vi "TraverseDoAllChannels.vi"(0 "Current Pulses positions for all channels":sgl[](array[numeric]), 1 "Current Pos In Eng units of all channels":sgl[](array[numeric]) format="%.2f", 2 "Counters Reset?":bool, 5 "Backlash Compensation?":bool, 7 "Home":T1, 9 "Mode":T5, 11 "Position Steps":sgl[][](array[numeric]) format="%.2f", 12 "Matched Configurations all Channels In":T2[](array[typedef]) {"Static Drive Configuration"."Indexer Mode  (FSA)" items=["Incremental", "Absolute"]; "Static Drive Configuration"."Buffer at Stop (SSH)" items=["Clear buffer", "Save and Continue"]; "Static Drive Configuration"."Buffer at Limit (SSG)" items=["Clear buffer", "Save and Continue"]; "Static Drive Configuration"."RS232 Echo Control (SSA)" items=["Echo ON", "Echo OFF"]; "Static Drive Configuration"."Reference edge of Home (OSH)" items=["CW", "CCW"]; "Static Drive Configuration"."Encoder Z for Home (OSD)" items=["Don't use", "Enable"]; "Static Drive Configuration"."Home Switch Sense (OSC)" items=["Normally Open", "Normally Closed"]; "Static Drive Configuration"."Home Position (OSB)" items=["Anywhere in Switch", "Edge of Switch"]; "Static Drive Configuration"."Limit Switch Sense (OSA)" items=["Normally Closed", "Normally Open"]; "Static Drive Configuration"."Limit Disable (LD)" items=["Both Enabled", "CW Disabled", "CCW Disabled", "Both Disabled"]; "Static Drive Configuration"."Stall Detect (FSH)" items=["Disable", "Enable"]; "Static Drive Configuration"."OP2 in Deadband (FSG)" items=["Don't Use", "ACTIVATE"]; "Static Drive Configuration"."Stop on Trigger 3 (FSF)" items=["Ignore", "STOP!"]; "Static Drive Configuration"."Activate OP1 on stall (FSE)" items=["Do not Activate", "ACTIVATE!"]; "Static Drive Configuration"."Stop on Stall (FSD)" items=["Continue", "STOP"]; "Static Drive Configuration"."Position Maintenance (FSC)" items=["Disabled", "Enabled"]; "Static Drive Configuration"."Step Mode  (FSB)" items=["Motor", "Encoder"]; "Static Drive Configuration"."Encoder Resolution (ER)" min=1 max=50000; "Static Drive Configuration"."Dead Band Window (DW)" min=0 max=999999999; "Static Drive Configuration"."Dead Band (DB)" min=0 max=999999999; "Static Drive Configuration"."Correction Gain % (CG)" items=["n/a", "12.5", "25", "37.5", "50", "62.5", "75", "87.5", "100"]; "Channel Properties"."Current Pos" format="%.2f"; "Channel Properties"."Backlash/Eng units" format="%.2f"; "Channel Properties"."Pulses/rev" format="%.2f"; "Channel Properties"."Pos Tolerance" format="%.2f"; "Channel Properties"."Pulses/unit" format="%.2f"; "Channel Properties"."Acc. Min" format="%.2f"; "Channel Properties"."Acc. Max" format="%.2f"; "Channel Properties"."Vel. Min" format="%.2f"; "Channel Properties"."Vel. Max" format="%.2f"; "Channel Properties"."Acc. Default" format="%.2f"; "Channel Properties"."Vel. Default" format="%.2f"}, 13 "Last Part of Move?":bool, 14 "Traverse Name":string="EnFlo Tunnel") -> (4 "Achieved Pos In Eng units of all channels":sgl[](array[numeric]) format="%.2f", 6 "Current Pulses positions for all channels Out":sgl[](array[numeric]), 8 "Moved?":bool, 10 "Error String":string, 15 "Matched Configurations Out":T2[](array[typedef]) {"Static Drive Configuration"."Indexer Mode  (FSA)" items=["Incremental", "Absolute"]; "Static Drive Configuration"."Buffer at Stop (SSH)" items=["Clear buffer", "Save and Continue"]; "Static Drive Configuration"."Buffer at Limit (SSG)" items=["Clear buffer", "Save and Continue"]; "Static Drive Configuration"."RS232 Echo Control (SSA)" items=["Echo ON", "Echo OFF"]; "Static Drive Configuration"."Reference edge of Home (OSH)" items=["CW", "CCW"]; "Static Drive Configuration"."Encoder Z for Home (OSD)" items=["Don't use", "Enable"]; "Static Drive Configuration"."Home Switch Sense (OSC)" items=["Normally Open", "Normally Closed"]; "Static Drive Configuration"."Home Position (OSB)" items=["Anywhere in Switch", "Edge of Switch"]; "Static Drive Configuration"."Limit Switch Sense (OSA)" items=["Normally Closed", "Normally Open"]; "Static Drive Configuration"."Limit Disable (LD)" items=["Both Enabled", "CW Disabled", "CCW Disabled", "Both Disabled"]; "Static Drive Configuration"."Stall Detect (FSH)" items=["Disable", "Enable"]; "Static Drive Configuration"."OP2 in Deadband (FSG)" items=["Don't Use", "ACTIVATE"]; "Static Drive Configuration"."Stop on Trigger 3 (FSF)" items=["Ignore", "STOP!"]; "Static Drive Configuration"."Activate OP1 on stall (FSE)" items=["Do not Activate", "ACTIVATE!"]; "Static Drive Configuration"."Stop on Stall (FSD)" items=["Continue", "STOP"]; "Static Drive Configuration"."Position Maintenance (FSC)" items=["Disabled", "Enabled"]; "Static Drive Configuration"."Step Mode  (FSB)" items=["Motor", "Encoder"]; "Static Drive Configuration"."Encoder Resolution (ER)" min=1 max=50000; "Static Drive Configuration"."Dead Band Window (DW)" min=0 max=999999999; "Static Drive Configuration"."Dead Band (DB)" min=0 max=999999999; "Static Drive Configuration"."Correction Gain % (CG)" items=["n/a", "12.5", "25", "37.5", "50", "62.5", "75", "87.5", "100"]; "Channel Properties"."Current Pos" format="%.2f"; "Channel Properties"."Backlash/Eng units" format="%.2f"; "Channel Properties"."Pulses/rev" format="%.2f"; "Channel Properties"."Pos Tolerance" format="%.2f"; "Channel Properties"."Pulses/unit" format="%.2f"; "Channel Properties"."Acc. Min" format="%.2f"; "Channel Properties"."Acc. Max" format="%.2f"; "Channel Properties"."Vel. Min" format="%.2f"; "Channel Properties"."Vel. Max" format="%.2f"; "Channel Properties"."Acc. Default" format="%.2f"; "Channel Properties"."Vel. Default" format="%.2f"})   [LabVIEW 2017]
uses:
  Anemometry/Anemometry Sub Vis/Gen Trav/Trav_mode.ctl
  ~subVIs/AxisConfigCluster.ctl
  ~subVIs/DriveProperties.ctl
  ~subVIs/DriveStaticConfig.ctl
  Anemometry/Anemometry Sub Vis/Controls/Home.ctl
  ~subVIs/DriveGotoCluster.ctl
  ~subVIs/DriveConfigGlobal.vi
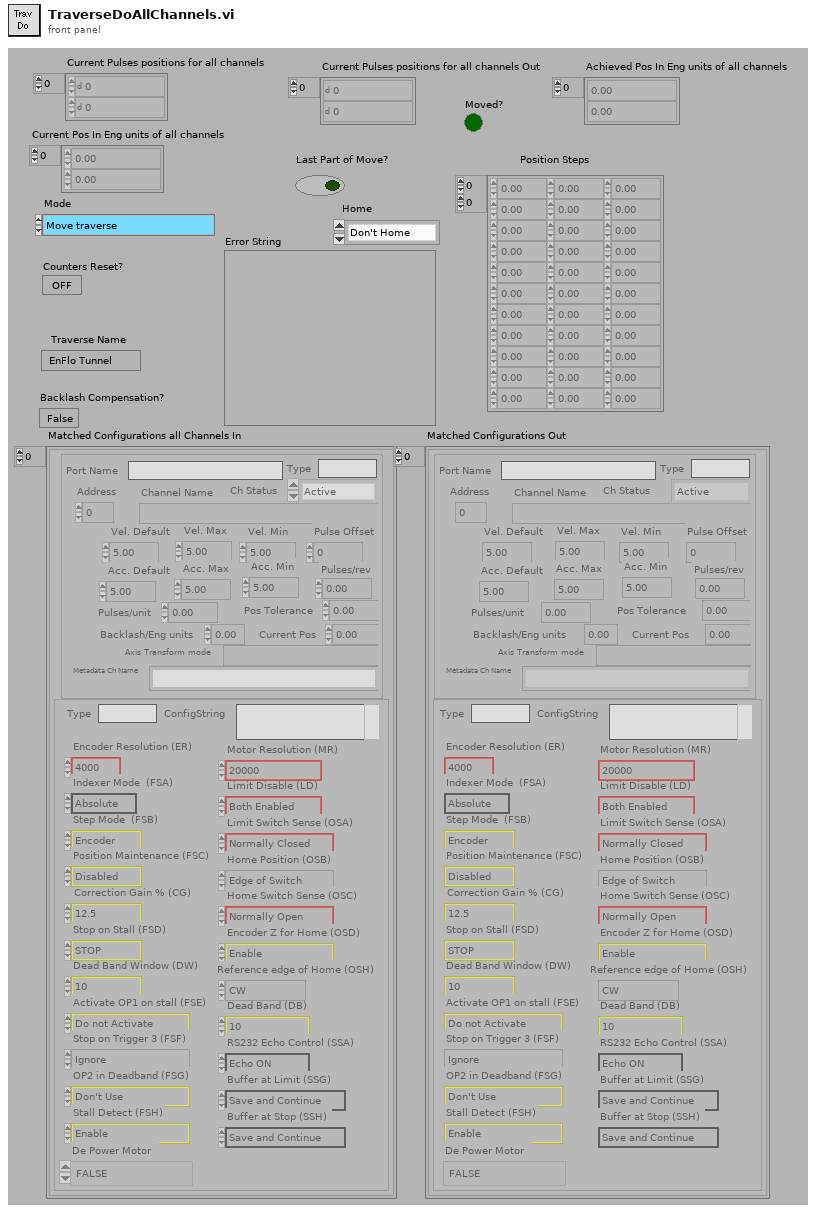
[diagram p1: front panel]
types:
  T1 = typedef "Home.ctl" = enum16{"Don't Home", "Home  +X", "Home  -X", "Home  +Y", "Home  -Y", "Home  +Z", "Home  -Z"}
  T2 = typedef "AxisConfigCluster.ctl" = cluster{"Channel Properties":T3, "Static Drive Configuration":T4}
  T3 = typedef "DriveProperties.ctl" = cluster{"Channel Name":string, "Vel. Default":sgl, "Acc. Default":sgl, "Vel. Max":sgl, "Vel. Min":sgl, "Acc. Max":sgl, "Acc. Min":sgl, "Pulses/unit":sgl, "Address":u8, "Pulse Offset":i32, "Pos Tolerance":sgl, "Pulses/rev":sgl, "Backlash/Eng units":sgl, "Current Pos":sgl, "Ch Status":enum16{"Active", "Offline", "Simulate"}, "Port Name":string, "Axis Transform mode":string, "Metadata Ch Name":string, "Type":string}
  T4 = typedef "DriveStaticConfig.ctl" = cluster{"Correction Gain % (CG)":u16, "Dead Band (DB)":i32, "Dead Band Window (DW)":i32, "Encoder Resolution (ER)":i32, "Step Mode  (FSB)":u16, "Position Maintenance (FSC)":u16, "Stop on Stall (FSD)":u16, "Activate OP1 on stall (FSE)":u16, "Stop on Trigger 3 (FSF)":u16, "OP2 in Deadband (FSG)":u16, "Stall Detect (FSH)":u16, "Limit Disable (LD)":u16, "Motor Resolution (MR)":enum16{"200", "400", "1000", "2000", "4000", "5000", "10000", "12800", "18000", "20000", "21600", "25000", "25400", "25600", "36000", "50000", "278528", "425984", "507904", "614400", "655360", "819200", "1024000"}, "Limit Switch Sense (OSA)":u16, "Home Position (OSB)":u16, "Home Switch Sense (OSC)":u16, "Encoder Z for Home (OSD)":u16, "Reference edge of Home (OSH)":u16, "RS232 Echo Control (SSA)":u16, "Buffer at Limit (SSG)":u16, "Buffer at Stop (SSH)":u16, "Indexer Mode  (FSA)":u16, "Type":string, "ConfigString":string, "De Power Motor":enum16{"TRUE", "FALSE"}}
  T5 = typedef "Trav_mode.ctl" = enum16{"Move traverse", "Read traverse position", "Teach Position"}
  T6 = enum16{"Load setup from excel file", "Save setup to excel file"}
  T7 = typedef "DriveGotoCluster.ctl" = cluster{"Channel name":string, "Go To Position":dbl}
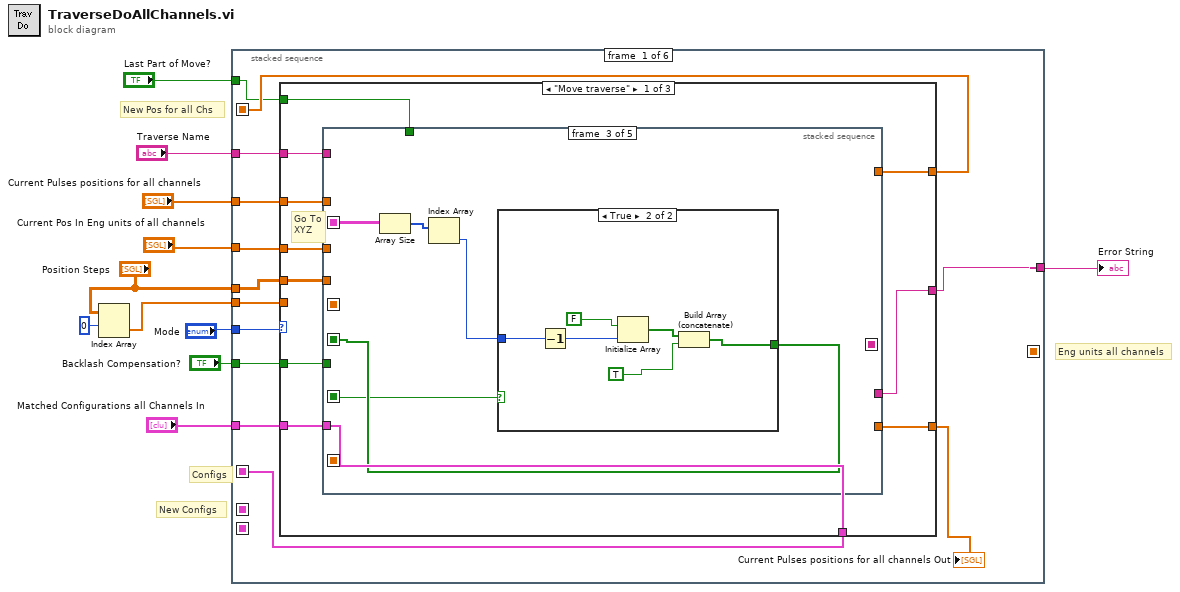
[diagram p0: block diagram]
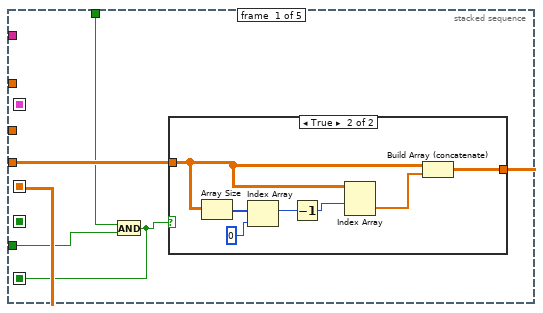
[diagram p2: hidden frame]
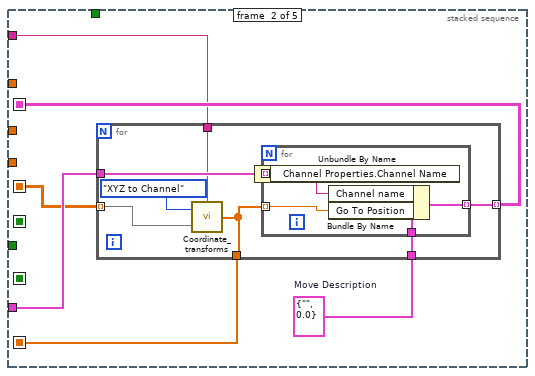
[diagram p4: hidden frame]
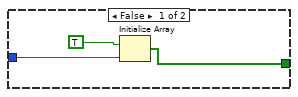
[diagram p5: hidden frame]
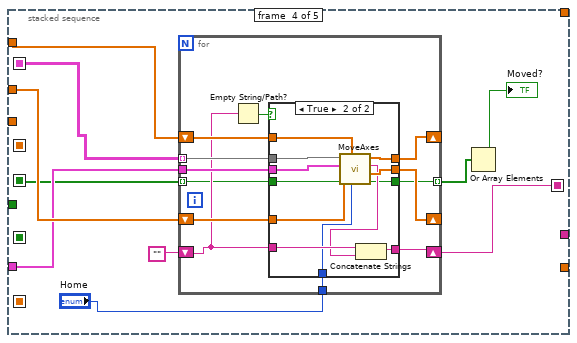
[diagram p6: hidden frame]
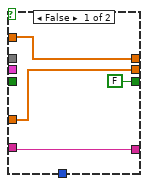
[diagram p7: hidden frame]
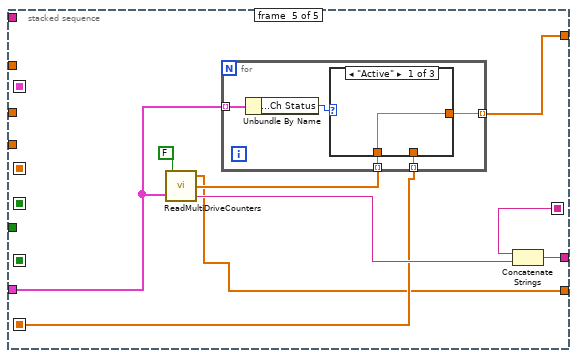
[diagram p8: hidden frame]
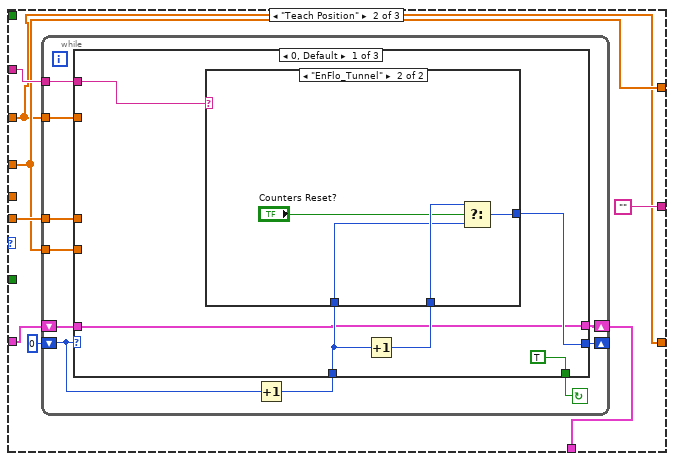
[diagram p11: hidden frame]
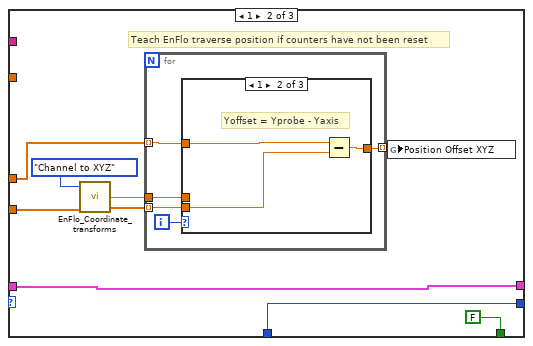
[diagram p13: hidden frame]
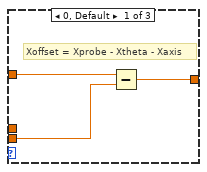
[diagram p14: hidden frame]
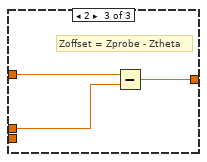
[diagram p15: hidden frame]
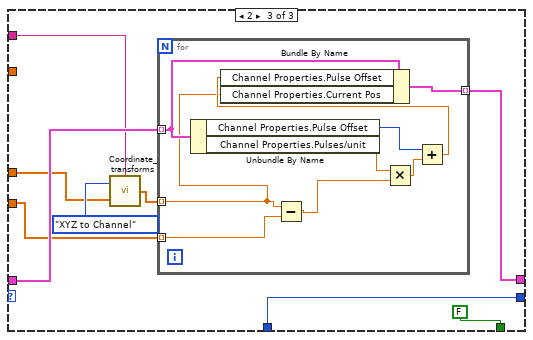
[diagram p16: hidden frame]
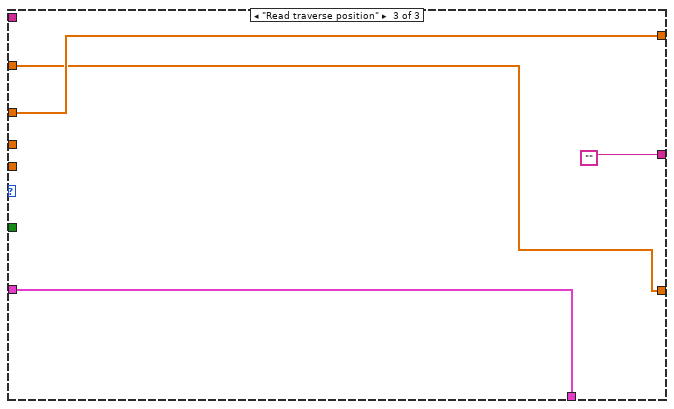
[diagram p17: hidden frame]
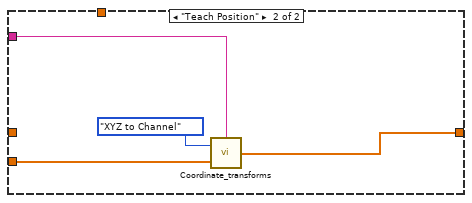
[diagram p19: hidden frame]
diagram:
  # "New Pos for all Chs"
  # "Eng units all channels"
  # "New Configs"
  # "Configs"
  n1 = Index Array(array="Position Steps", index (row)=0 ("Index")) -> (element=w2:sgl[])  [unwired: 1 in]
  n2 = stacked-sequence {
    seq-local: [_ w212 _ _ _ _] -> [_ _ _ w221 _ _]
    seq-local: [w23 _ _ _ _ _] -> [_ _ _ w223 _ _]
    seq-local: [_ _ _ w222 _ _] -> [_ _ _ _ w230 _]
    seq-local: [w14 _ _ _ _ _] -> [_ w209 _ _ _ _]
    seq-local: [_ _ _ _ w228 _] -> [_ _ _ _ _ w237]
    tunnel: "Mode" -> [w24 w213 _ _ _ w238]
    tunnel: "Current Pos In Eng units of all channels" -> [w21 w214 _ _ _ _]
    tunnel: "Matched Configurations all Channels In" -> [w22 _ _ _ _ _]
    tunnel: "Current Pulses positions for all channels" -> [w20 _ _ _ _ _]
    tunnel: [w19 _ _ _ _ _] -> w7
    tunnel: "Traverse Name" -> [w18 w211 _ _ w229 w236]
    tunnel: "Position Steps" -> [w17 _ _ _ _ _]
    tunnel: "Backlash Compensation?" -> [w16 _ _ _ _ _]
    tunnel: w2 -> [w15 w210 _ _ _ _]
    tunnel: "Last Part of Move?" -> [w12 _ w220 _ w227 _]
    frame #0 {
      n3 = case shown="\"Move traverse\"" w24 {
        tunnel: [w34 w139 w208] -> w23
        tunnel: w22 -> [w34 w140 w208]
        tunnel: w21 -> [w32 w136 w206]
        tunnel: w20 -> [w33 w135 w205]
        tunnel: [w31 "" ""] -> w19
        tunnel: w18 -> [w29 w141 _]
        tunnel: w17 -> [w30 _ _]
        tunnel: w16 -> [w28 _ _]
        tunnel: w15 -> [_ w137 _]
        tunnel: [w27 w136 w206] -> w14
        tunnel: [w26 w135 w205] -> w13
        tunnel: w12 -> [w25 _ _]
        frame "Move traverse" {
          # "Go To\nXYZ"
          n4 = stacked-sequence {
            seq-local: [_ w51 _ _ _] -> [_ _ w70 w86 _]
            seq-local: [w39 _ _ _ _] -> [_ w50 _ _ _]
            seq-local: [_ _ _ w84 _] -> [_ _ _ _ w125]
            seq-local: [_ w48 _ _ _] -> [_ _ _ _ w119]
            seq-local: [w35 _ _ _ _] -> [_ _ w66 _ _]
            seq-local: [_ _ w69 _ _] -> [_ _ _ w80 _]
            tunnel: w34 -> [_ w52 _ w85 w122]
            tunnel: w33 -> [_ _ _ w89 _]
            tunnel: w32 -> [_ _ _ w88 _]
            tunnel: [_ _ _ _ w123] -> w31
            tunnel: w30 -> [w38 _ _ _ _]
            tunnel: w29 -> [_ w49 _ _ _]
            tunnel: w28 -> [w37 _ _ _ _]
            tunnel: [_ _ _ _ w121] -> w27
            tunnel: [_ _ _ _ w118] -> w26
            tunnel: w25 -> [w36 _ _ _ _]
            frame #0 {
              n5 = And(x=w36, y=w37) -> (x .and. y?=w35:bool)
              n6 = case shown="True" w35 {
                tunnel: w38 -> [w40 w42]
                tunnel: [w40 w41] -> w39
                frame False {
                }
                frame True {
                  n7 = Array Size(array=w42) -> (size(s)=w47:i32[])
                  n8 = Index Array(array=w47, index=0 ("Index")) -> (element=w45:i32)
                  n9 = Decrement(x=w45) -> (x-1=w44:i32)
                  n10 = Index Array(array=w42, index (row)=w44) -> (element=w43:sgl[])  [unwired: 1 in]
                  n11 = Build Array (concatenate)(w42, w43) -> (w41:sgl[][])
                }
              }
            }
            frame #1 {
              w53 = T7 {"Channel name"="", "Go To Position"=0.0}  # Move Description
              n12 = for {
                tunnel: w53 -> [w60]
                tunnel: w52 -> [w59]
                tunnel: [w58] -> w51 mode=indexing
                tunnel: w50 -> [w55] mode=indexing
                tunnel: w49 -> [w56]
                tunnel: [w54] -> w48
                n13 = call "Coordinate_transforms.vi"("Traverse Name"=w56, "Input"=w55, "Mode"=enum16{"XYZ to Channel", "Channel to XYZ"}."XYZ to Channel") -> ("Output"=w54:sgl[])
                n14 = for {
                  tunnel: w54 -> [w65] mode=indexing
                  tunnel: [w64] -> w58 mode=indexing
                  tunnel: w59 -> [w62] mode=indexing
                  tunnel: w60 -> [w61]
                  n15 = Unbundle By Name(w62) -> ("Channel Properties.Channel Name"=w63:string)
                  n16 = Bundle By Name(cluster=w61, "Channel name"=w63, "Go To Position"=w65) -> (w64:T7)
                }
              }
            }
            frame #2 {
              n17 = Array Size(array=w70) -> (size(s)=w68:i32[])
              n18 = Index Array(array=w68) -> (element=w67:i32)  [unwired: 1 in]
              n19 = case shown="True" w66 {
                tunnel: [w71 w79] -> w69
                tunnel: w67 -> [w72 w77]
                frame False {
                  n20 = Initialize Array(TRUE, w72) -> (w71:bool[])
                }
                frame True {
                  n21 = Decrement(x=w77) -> (x-1=w78:i32)
                  n22 = Initialize Array(FALSE, w78) -> (w75:bool[])
                  n23 = Build Array (concatenate)(w75, TRUE) -> (w79:bool[])
                }
              }
            }
            frame #3 {
              n24 = for {
                tunnel: w86 -> [w101] mode=indexing
                tunnel: w85 -> [w100]
                shift-right: [w97] -> _
                shift-left: w89 -> [w96]
                shift-right: [w98] -> _
                shift-left: w88 -> [w99]
                shift-right: [w95] -> w84
                shift-left: "" -> [w94]
                tunnel: "Home" -> [w92]
                tunnel: [w91] -> w82 mode=indexing
                tunnel: w80 -> [w90] mode=indexing
                n25 = Empty String/Path?(string/path=w94) -> (empty?=w93:bool)
                n26 = case shown="True" w93 {
                  tunnel: w101 -> [_ w117]
                  tunnel: w100 -> [_ w116]
                  tunnel: w99 -> [w104 w115]
                  tunnel: [w104 w114] -> w98
                  tunnel: [w105 w113] -> w97
                  tunnel: w96 -> [w105 w112]
                  tunnel: [w103 w109] -> w95
                  tunnel: w94 -> [w103 w111]
                  tunnel: w92 -> [_ w108]
                  tunnel: [FALSE ("Moved?") w107] -> w91
                  tunnel: w90 -> [_ w106]
                  frame False {
                  }
                  frame True {
                    n27 = call "MoveAxes.vi"("Home"=w108, "Current Pulses In"=w112, "Pos without backlash"=w106, "Current Pos In"=w115, "Matched Configurations"=w116, "GoTo Array (Eng units all channels)"=w117) -> ("Moved?"=w107:bool, "Current Pos Out"=w114:dbl[], "Error String"=w110:string, "Current Pulses Out"=w113:dbl[])
                    n28 = Concatenate Strings(w111, w110) -> (w109:string)
                  }
                }
              }
              n29 = Or Array Elements(Boolean array=w82) -> (logical OR=→"Moved?":bool)
            }
            frame #4 {
              n30 = call "ReadMultiDriveCounters.vi"("Recheck if Moved?"=FALSE, "Matched Configurations"=w122) -> ("Pulses"=w118:sgl[], "Eng units"=w120:sgl[], "Error String"=w124:string)
              n31 = for {
                tunnel: w122 -> [w131] mode=indexing
                tunnel: [w129] -> w121 mode=indexing
                tunnel: w120 -> [w128] mode=indexing
                tunnel: w119 -> [w127] mode=indexing
                n32 = Unbundle By Name(w131) -> ("Channel Properties.Ch Status"=w130:enum16{"Active", "Offline", "Simulate"})
                n33 = case shown="\"Active\"" w130 {
                  tunnel: [w132 w133 w134] -> w129
                  tunnel: w128 -> [w132 _ w134]
                  tunnel: w127 -> [_ w133 _]
                  frame "Active" {
                  }
                  frame "Simulate" {
                  }
                  frame "Offline" {
                  }
                }
              }
              n34 = Concatenate Strings(w125, w124) -> (w123:string)
            }
          }
        }
        frame "Teach Position" {
          n35 = while {
            tunnel: w137 -> [w143]
            shift-left: w140 -> [w145]
            shift-right: [w144] -> w139
            tunnel: w136 -> [w146]
            tunnel: w135 -> [w147]
            tunnel: w141 -> [w148]
            shift-left: 0 -> [w152]
            shift-right: [w149] -> _
            stop <- w151 continue-if-true
            n36 = Increment(x=w152) -> (x+1=w150:i32)
            n37 = case shown="0, Default" w152 {
              tunnel: [TRUE FALSE FALSE] -> w151
              tunnel: w150 -> [w155 w166 w195]
              tunnel: [w156 w166 w195] -> w149
              tunnel: w148 -> [w157 _ w188]
              tunnel: w147 -> [_ _ _]
              tunnel: w146 -> [_ w167 w189]
              tunnel: w145 -> [w153 w165 w193]
              tunnel: [w153 w165 w192] -> w144
              tunnel: w143 -> [_ w164 w187]
              frame 0, Default {
                n38 = Increment(x=w155) -> (x+1=w154:i32)
                n39 = case shown="\"EnFlo_Tunnel\"" w157 {
                  tunnel: [w159 w163] -> w156
                  tunnel: w155 -> [_ w161]
                  tunnel: w154 -> [w159 w162]
                  frame "A_Tunnel", Default {
                  }
                  frame "EnFlo_Tunnel" {
                    n40 = Select(t=w162, s="Counters Reset?", f=w161) -> (s? t:f=w163:i32)
                  }
                }
              }
              frame 1 {
                # "Teach EnFlo traverse position if counters have not been reset"
                n41 = call "EnFlo_Coordinate_transforms.vi"("Input"=w167, "Mode"=enum16{"XYZ to Channel", "Channel to XYZ"}."Channel to XYZ") -> ("Output"=w170:dbl[], "Z theta"=w169:dbl)  [unwired: 2 out]
                n42 = for {
                  tunnel: w164 -> [w176] mode=indexing
                  tunnel: w170 -> [w175] mode=indexing
                  tunnel: [w174] -> w171 mode=indexing
                  tunnel: w169 -> [w173]
                  i -> [w177]
                  n43 = case shown="1" w177 {
                    tunnel: w176 -> [w180 w183 w186]
                    tunnel: w175 -> [w179 w182 _]
                    tunnel: [w178 w181 w184] -> w174
                    tunnel: w173 -> [_ _ w185]
                    frame 0, Default {
                      # "Xoffset = Xprobe - Xtheta - Xaxis"
                      n44 = Subtract(x=w180, y=w179) -> (x-y=w178:dbl)
                    }
                    frame 1 {
                      # "Yoffset = Yprobe - Yaxis"
                      n45 = Subtract(x=w183, y=w182) -> (x-y=w181:dbl)
                    }
                    frame 2 {
                      # "Zoffset = Zprobe - Ztheta"
                      n46 = Subtract(x=w186, y=w185) -> (x-y=w184:dbl)
                    }
                  }
                }
                n47 = global write "DriveConfigGlobal.vi" "Position Offset XYZ"(w171) -> ()
              }
              frame 2 {
                n48 = call "Coordinate_transforms.vi"("Traverse Name"=w188, "Input"=w187, "Mode"=enum16{"XYZ to Channel", "Channel to XYZ"}."XYZ to Channel") -> ("Output"=w190:sgl[])
                n49 = for {
                  tunnel: w193 -> [w204] mode=indexing
                  tunnel: [w202] -> w192 mode=indexing
                  tunnel: w189 -> [w200] mode=indexing
                  tunnel: w190 -> [w196] mode=indexing
                  n50 = Unbundle By Name(w204) -> ("Channel Properties.Pulse Offset"=w201:i32, "Channel Properties.Pulses/unit"=w199:sgl)
                  n51 = Subtract(x=w196, y=w200) -> (x-y=w197:sgl)
                  n52 = Multiply(x=w199, y=w197) -> (x*y=w198:sgl)
                  n53 = Add(x=w201, y=w198) -> (x+y=w203:sgl)
                  n54 = Bundle By Name(cluster=w204, "Channel Properties.Pulse Offset"=w203, "Channel Properties.Current Pos"=w196) -> (w202:T2)
                }
              }
            }
          }
        }
        frame "Read traverse position" {
        }
      }
      "Current Pulses positions for all channels Out" <- w13
    }
    frame #1 {
      # "Eng units all channels"
      n55 = case shown="\"Move traverse\", Default" w213 {
        tunnel: w214 -> [_ _]
        tunnel: [w215 w218] -> w212
        tunnel: w211 -> [_ w217]
        tunnel: w210 -> [_ w216]
        tunnel: w209 -> [w215 _]
        frame "Move traverse", Default {
        }
        frame "Teach Position" {
          n56 = call "Coordinate_transforms.vi"("Traverse Name"=w217, "Input"=w216, "Mode"=enum16{"XYZ to Channel", "Channel to XYZ"}."XYZ to Channel") -> ("Output"=w218:sgl[])
        }
      }
    }
    frame #2 {
      n57 = case shown="False" w220 {
        frame False {
        }
        frame True {
          n58 = call "Shut_down_all_Axis.vi"() -> ()  [unwired: 1 out]
        }
      }
    }
    frame #3 {
      n59 = for {
        tunnel: [w226] -> w222 mode=indexing
        tunnel: w223 -> [w225] mode=indexing
        tunnel: w221 -> [w224] mode=indexing
        n60 = Bundle By Name(cluster=w225, "Channel Properties.Current Pos"=w224) -> (w226:T2)
      }
      "Achieved Pos In Eng units of all channels" <- w221
    }
    frame #4 {
      n61 = case shown="True" w227 {
        tunnel: w230 -> [w231 w234]
        tunnel: w229 -> [_ w233]
        tunnel: [w231 w232] -> w228
        frame False {
        }
        frame True {
          n62 = call "Read_Write_Trav_position.vi"("Matched Configurations In"=w234, "Mode"=T6."Save setup to excel file", "Traverse Name"=w233) -> ("Matched Configurations Out"=w232:T2[])  [unwired: 1 out]
        }
      }
      "Matched Configurations Out" <- w228
    }
    frame #5 {
      n63 = case shown="\"Move traverse\", Default" w238 {
        tunnel: w237 -> [_ w240]
        tunnel: w236 -> [_ w239]
        frame "Move traverse", Default {
        }
        frame "Teach Position" {
          n64 = stacked-sequence {
            tunnel: w240 -> [w243 _]
            tunnel: w239 -> [_ w253]
            frame #0 {
              n65 = global read "DriveConfigGlobal.vi" "Configurations"() -> (w242:T2[])
              n66 = for {
                tunnel: w242 -> [w252] mode=indexing
                tunnel: [w251] -> w244 mode=indexing
                n67 = Unbundle By Name(w252) -> ("Channel Properties.Channel Name"=w251:string)
              }
              n68 = for {
                tunnel: w244 -> [w250]
                tunnel: w243 -> [w245] mode=indexing
                shift-right: [w247] -> w241
                shift-left: w242 -> [w248]
                n69 = Unbundle By Name(w245) -> ("Channel Properties.Channel Name"=w249:string)
                n70 = Search 1D Array(1D array=w250, element=w249) -> (index of element=w246:i32)  [unwired: 1 out]
                n71 = Replace Array Subset(array=w248, new element=w245, index=w246) -> (w247:T2[])
              }
              n72 = global write "DriveConfigGlobal.vi" "Configurations"(w241) -> ()
            }
            frame #1 {
              n73 = call "Read_Write_Trav_Config.vi"("Traverse Name"=w253, "Mode"=T6."Save setup to excel file") -> ()  [unwired: 1 out]
            }
          }
        }
      }
    }
  }
  "Error String" <- w7
